vi "Add Buffer Data to Variant.vi"(8 "error in (no error)":errorcluster, 9 "Buffer data":T1, 10 "tag":string, 11 "Application Data In in":T2) -> (0 "error out":errorcluster, 3 "Application Data In out":T2)   [LabVIEW 2017, in "DSF Data Viewer.lvlib"]
uses:
  DSF Data Viewer.lvlib
  Main VI/Application Data.ctl
  Builds/Data Sharing Framework/Current/Core/DSF Core.lvlibp/Engine/Classes/Framework/Framework.lvclass
  <vilib>/NI/Memory Manager/Classes/Pointer/Pointer.lvclass
  Buffer Reader/Buffer Data.ctl
  Builds/Data Sharing Framework/Current/Core/DSF Core.lvlibp/Engine/Classes/Buffer/Buffer.lvclass
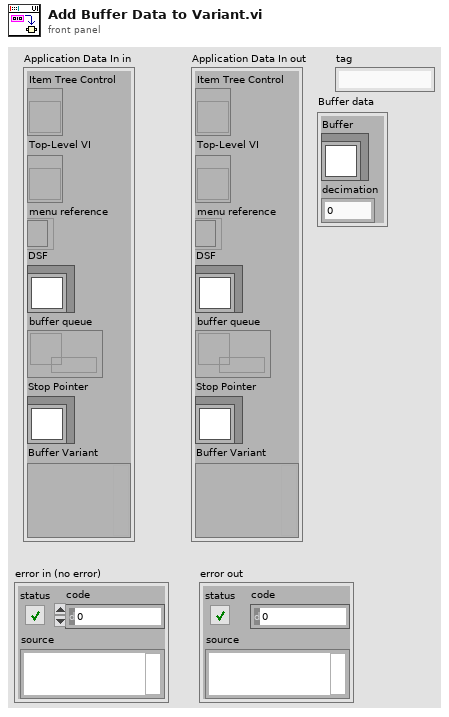
[diagram p1: front panel]
types:
  T1 = typedef "DSF Data Viewer.lvlib/Buffer Data.ctl" = cluster{"Buffer":refnum<class "Buffer.lvclass">, "decimation":u64}
  T2 = typedef "DSF Data Viewer.lvlib/Application Data.ctl" = cluster{"Item Tree Control":refnum<vi>, "Top-Level VI":refnum<vi>, "menu reference":refnum<k9>, "DSF":refnum<class "Framework.lvclass">, "buffer queue":refnum<queue>, "Stop Pointer":refnum<class "Pointer.lvclass">, "Buffer Variant":variant}
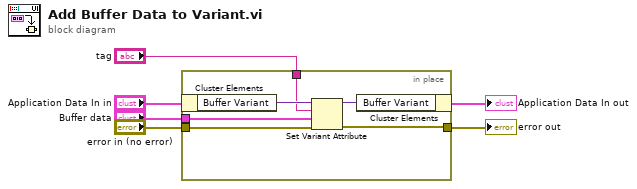
[diagram p0: block diagram]
diagram:
  n1 = in-place {
    in-place-border: [w10] -> w3
    in-place-border: "error in (no error)" -> [w11]
    in-place-border: "tag" -> [w9]
    in-place-border: "Buffer data" -> [w7]
    n2 = in-place-cluster #1("Application Data In in") -> ("Buffer Variant"=w12:variant)
    n3 = Set Variant Attribute(Variant=w12, name=w9, value=w7, error in=w11) -> (Variant out=w8:variant, error out=w10:errorcluster)  [unwired: 1 out]
    n4 = in-place-cluster #1("Buffer Variant"=w8) -> (→"Application Data In out":T2)
  }
  "error out" <- w3
